vi "Has focus actor.vi"(10 "user event in":refnum<user-event>, 11 "Control Ref":refnum<vi>) -> ()   [LabVIEW 2023]
doc: "Monitor control for key focus status at 10Hz until control ref becomes invalid.\n\n(Would it be better to monitor if the calling VI is running? Assume this is only used on a user interface.\n\nVI is reentrant, so you can monitor as many controls as you want."
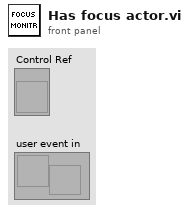
[diagram p1: front panel]
types:
  T1 = cluster{"Control Ref":refnum<vi>, "Key Focus":bool}
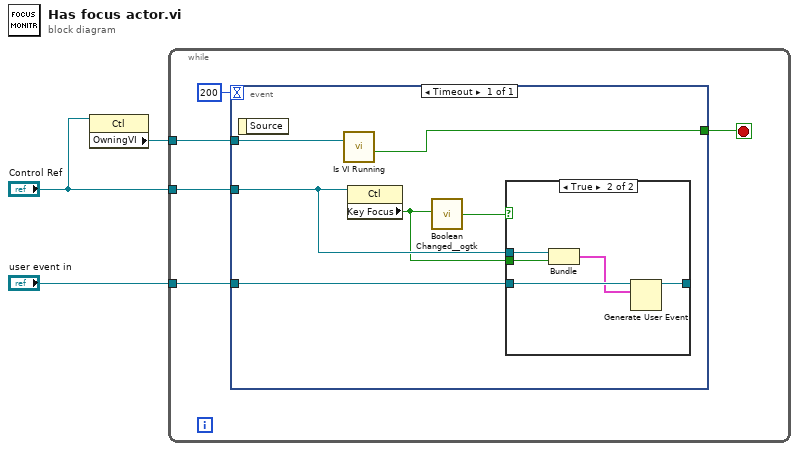
[diagram p0: block diagram]
diagram:
  n1 = property class="Ctl"(reference="Control Ref") -> ("OwningVI"=w1:refnum<vi>)  [unwired: 1 in, 2 out]
  n2 = while {
    tunnel: "Control Ref" -> [w8]
    tunnel: "user event in" -> [w7]
    tunnel: w1 -> [w5]
    stop <- w4 stop-if-true
    n3 = event shown="[0] Timeout" {
      selector: _ -> [_]
      dyn-events: _ -> [_]
      timeout: 200 -> [_]
      tunnel: w8 -> [w12]
      tunnel: w7 -> [w14]
      tunnel: [w9] -> w4
      tunnel: w5 -> [w10]
      event Timeout {
        n4 = event-data() -> ()  [unwired: 1 in, 1 out]
        n5 = call "Is VI Running.vi"("VI in"=w10) -> ("VI Not Running"=w9:bool)  [unwired: 7 in, 3 out]
        n6 = property class="Ctl"(reference=w12) -> ("Key Focus"=w11:bool)  [unwired: 1 in, 2 out]
        n7 = call <userlib>:"Boolean Changed__ogtk.vi"("Boolean"=w11) -> ("Changed"=w13:bool)
        n8 = case shown="True" w13 {
          tunnel: w14 -> [w15 w20]
          tunnel: [w15 w19] -> _
          tunnel: w12 -> [_ w18]
          tunnel: w11 -> [_ w17]
          frame False {
          }
          frame True {
            n9 = Bundle("Control Ref"=w18, "Key Focus"=w17) -> (w16:T1)  [unwired: 1 in]
            n10 = Generate User Event(user event=w20, event data cluster=w16) -> (user event out=w19:refnum<user-event>)  [unwired: 2 in, 1 out]
          }
        }
      }
    }
  }
